vi "PH_PILS.ProcPeriodic.vi"(0 "i ref in":refnum<vi>, 3 "ms timeout (100)":i32=100, 5 "error in (no error)":errorcluster) -> (14 "i ref out":refnum<vi>, 17 "timed out":bool, 19 "error out":errorcluster)   [LabVIEW 2014, in "PH_PILS.lvlib"]
doc: "This method serves to periodically do things like reading values from the HW. Methods that should be executed periodically should be called from THIS methode. Add code here."
uses:
  PH_PILS.lvlib
  PH_Devices/PH_Beckhoff/PH_Beckhoff.lvlib
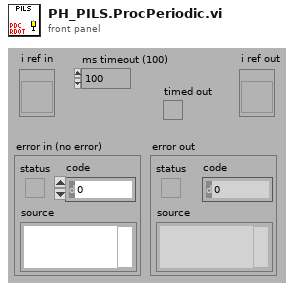
[diagram p1: front panel]
types:
  T1 = typedef "PH_PILS.lvlib/PH_PILS.i attribute.ctl" = cluster{"Boolean":cluster{"GUI Ref":refnum<vi>, "Status":i32}[], "GUI Refs Exp. Shutters":cluster{"1":refnum<vi>, "2":refnum<vi>, "3":refnum<vi>, "4":refnum<vi>}, "Tristate2Run GUI Refs":refnum<vi>[], "EO-Likes":cluster{"GUI Ref":refnum<vi>, "Status":i32}[], "Operation Mode":cluster{"Operation Mode":T2, "GUI":cluster{"Ref State":refnum<vi>, "Ref":refnum<vi>}, "Servicemode":cluster{"Tagname":string, "Status":i32}, "Labormode":cluster{"Tagname":string, "Status":i32}, "Searchmode":cluster{"Tagname":string, "Status":i32}, "Shotmode":cluster{"Tagname":string, "Status":i32}}, "Submode":cluster{"Submode":T3, "GUI":cluster{"Ref State":refnum<vi>, "Ref":refnum<vi>}, "Submode":cluster{"Tagname":string, "Status":i32}}, "Experiment":cluster{"Experiment":enum16{"unknown", "intern", "4 (Z6)", "3", "2", "1"}, "GUI":cluster{"Ref State":refnum<vi>, "Ref":refnum<vi>}, "intern":cluster{"Tagname":string, "Status":i32}, "Exp 4":cluster{"Tagname":string, "Status":i32}, "Exp 3":cluster{"Tagname":string, "Status":i32}, "Exp 2":cluster{"Tagname":string, "Status":i32}, "Exp 1":cluster{"Tagname":string, "Status":i32}}, "TristateNormal":cluster{"GUI Ref":refnum<vi>, "Status":i32}[], "Door Tags":cluster{"GUI Ref":refnum<vi>, "Status":i32}[], "GUIlessTags":cluster{"Name":string, "Status":i32}[], "Beamline GUI Refs":refnum<vi>[], "Special Boolean":cluster{"GUI Ref":refnum<vi>, "Status":i32}[], "Laserpower":cluster{"GUI Ref":refnum<vi>, "Status":i32}[], "Shutter":cluster{"GUI Ref":refnum<vi>, "Status":i32}[], "Tristate EO Like":cluster{"GUI Ref":refnum<vi>, "Status":i32}[], "PP":cluster{"GUI Ref":refnum<vi>, "Status":i32, "Head Ref":refnum<vi>, "Slider Ref":refnum<vi>}[], "Switch Knobs":cluster{"GUI Ref":refnum<vi>, "Status":i32}[], "Latch Knob GUI Refs":refnum<vi>[], "FailureCounter":i32, "Enabled Status":cluster{"Laser":i32, "PreAmp":i32, "MainAmp":i32}, "Mercury":refnum<vi>, "Instance Rods":string, "Logfile":path, "Beckhoff-Instance Internal":string, "Beckhoff-Instance External":string, "Enabling Rights":cluster{"Name":string, "Password":string, "PA?":bool, "MA?":bool, "Exp?":bool}[]}
  T2 = typedef "PH_PILS.lvlib/PH_PILS.Operation Mode.ctl" = enum16{"unknown", "Service", "Labor", "Search", "Shot"}
  T3 = typedef "PH_PILS.lvlib/PH_PILS.Submode.ctl" = enum16{"unknown", "HV-Normal", "HV-Test"}
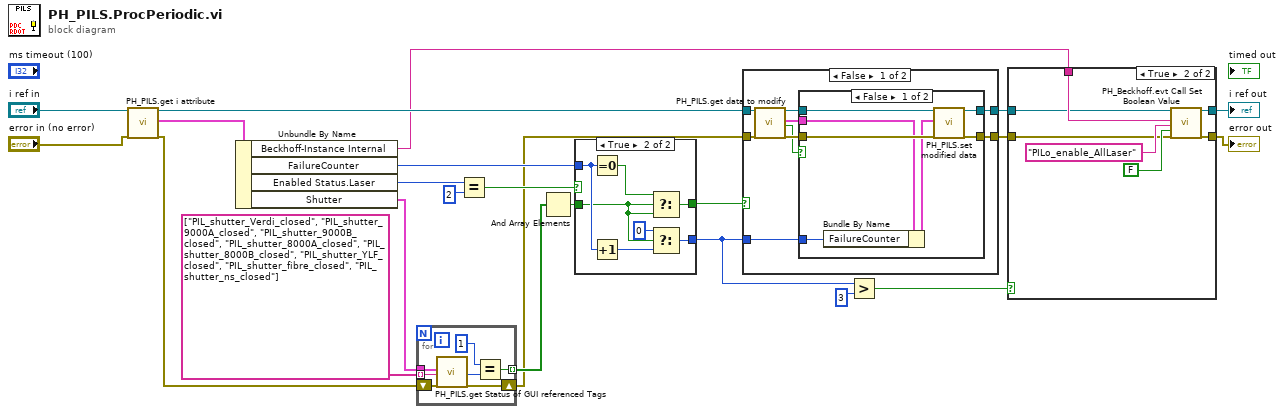
[diagram p0: block diagram]
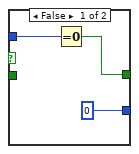
[diagram p5: hidden frame]
diagram:
  n1 = call "PH_PILS.get i attribute.vi"("i ref in"="i ref in", "error in (no error)"="error in (no error)") -> ("i ref out"=w15:refnum<vi>, "i attribute"=w22:T1, "error out"=w3:errorcluster)  [unwired: 15 in]
  n2 = Unbundle By Name(w22) -> ("Beckhoff-Instance Internal"=w1:string, "FailureCounter"=w16:i32, "Enabled Status.Laser"=w18:i32, "Shutter"=w20:cluster{"GUI Ref":refnum<vi>, "Status":i32}[])
  n3 = for {
    tunnel: w20 -> [w30]
    tunnel: string[] ["PIL_shutter_Verdi_closed", "PIL_shutter_9000A_closed", "PIL_shutter_9000B_closed", "PIL_shutter_8000A_closed", "PIL_shutter_8000B_closed", "PIL_shutter_YLF_closed", "PIL_shutter_fibre_closed", "PIL_shutter_ns_closed"] -> [w29] mode=indexing
    tunnel: [w27] -> w11 mode=indexing
    shift-right: [w24] -> w2
    shift-left: w3 -> [w28]
    n4 = call "PH_PILS.get Status of GUI referenced Tags.vi"("Tags"=w30, "Tagname"=w29, "error in"=w28) -> ("Status"=w26:i32, "error out"=w24:errorcluster)  [unwired: 13 in, 2 out]
    n5 = Equal?(x=1 ("y"), y=w26) -> (x = y?=w27:bool)
  }
  n6 = Equal?(x=w18, y=2) -> (x = y?=w13:bool)
  n7 = And Array Elements(Boolean array=w11) -> (logical AND=w10:bool)
  n8 = case shown="True" w13 {
    tunnel: w16 -> [w33 w36]
    tunnel: [w32 w39] -> w12
    tunnel: [0 ("FailureCounter") w38] -> w4
    tunnel: w10 -> [_ w34]
    frame False {
      n9 = Equal To 0?(x=w33) -> (x = 0?=w32:bool)
    }
    frame True {
      n10 = Equal To 0?(x=w36) -> (x = 0?=w40:bool)
      n11 = Increment(x=w36) -> (x+1=w35:i32)
      n12 = Select(t=w40, s=w34, f=w34) -> (s? t:f=w39:bool)
      n13 = Select(t=0 ("FailureCounter"), s=w34, f=w35) -> (s? t:f=w38:i32)
    }
  }
  n14 = case shown="False" w12 {
    tunnel: w15 -> [w48 w60]
    tunnel: [w47 w60] -> w9
    tunnel: w2 -> [w45 w59]
    tunnel: [w44 w59] -> w14
    tunnel: w4 -> [w41 _]
    frame False {
      n15 = call "PH_PILS.get data to modify.vi"("i ref in"=w48, "error in (no error)"=w45) -> ("i ref out"=w49:refnum<vi>, "i attribute"=w42:T1, "timed out"=w43:bool, "error out"=w46:errorcluster)  [unwired: 14 in]
      n16 = case shown="False" w43 {
        tunnel: w49 -> [w56 w58]
        tunnel: [w55 w58] -> w47
        tunnel: w46 -> [w54 w57]
        tunnel: [w53 w57] -> w44
        tunnel: w42 -> [w52 _]
        tunnel: w41 -> [w50 _]
        frame False {
          n17 = Bundle By Name(cluster=w52, "FailureCounter"=w50) -> (w51:T1)
          n18 = call "PH_PILS.set modified data.vi"("i ref in"=w56, "i attribute"=w51, "error in (no error)"=w54) -> ("i ref out"=w55:refnum<vi>, "error out"=w53:errorcluster)  [unwired: 15 in]
        }
        frame True {
        }
      }
    }
    frame True {
    }
  }
  n19 = Greater?(x=w4, y=3) -> (0:w5:bool)
  n20 = case shown="True" w5 {
    tunnel: w14 -> [w61 w63]
    tunnel: w9 -> [w62 w64]
    tunnel: [w61 w69] -> w8
    tunnel: [w62 w68] -> w7
    tunnel: w1 -> [_ w65]
    frame False {
    }
    frame True {
      n21 = call "PH_Beckhoff.evt Call Set Boolean Value.vi"("i ref in"=w64, "Beckhoff Instance"=w65, "Tagname to set"="PILo_enable_AllLaser", "Value"=FALSE ("Value to set"), "error in"=w63) -> ("i ref out"=w68:refnum<vi>, "error out"=w69:errorcluster)  [unwired: 13 in]
    }
  }
  "error out" <- w8
  "i ref out" <- w7
